vi "Test 2 Analog Sonar 3 MB7047 I2C Sensors.vi"() -> ()   [LabVIEW 2011]
uses:
  <vilib>/express/express arith-compare/Formula/XNode/ExpressFormulaBlockNode.xnode
  <vilib>/LabVIEW Interface for Arduino/LabVIEW Interface for Arduino.lvlib
panel:
  in  "Front Object\nDistance":i32=8
  out "Front Object":bool
  in  "Rear Object\nDistance":i32=3
  out "Rear Object":bool
  in  "Too Close\nto Manuver":i32=2
  out "Stop!":bool
  out "Turn Left":bool
  out "Right Front (ft)":dbl
  out "RF":dbl(slide) scale=0.0..10.0 scale format="%_4g"
  out "Left Front (ft)":dbl
  out "LF":dbl(slide) scale=0.0..10.0 scale format="%_4g"
  out "RB I2C Data":u8[](array[numeric]) format="%x"
  out "RB":u8(slide) scale=0.0..10.0
  out "Right Back (ft)":u32
  out "Center (ft)":u32
  out "C":u8(slide) scale=0.0..10.0
  out "C I2C Data":u8[](array[numeric]) format="%x"
  out "LB I2C Data":u8[](array[numeric]) format="%x"
  out "LB":u8(slide) scale=0.0..10.0
  out "Left Back (ft)":u32
  in  "stop":bool
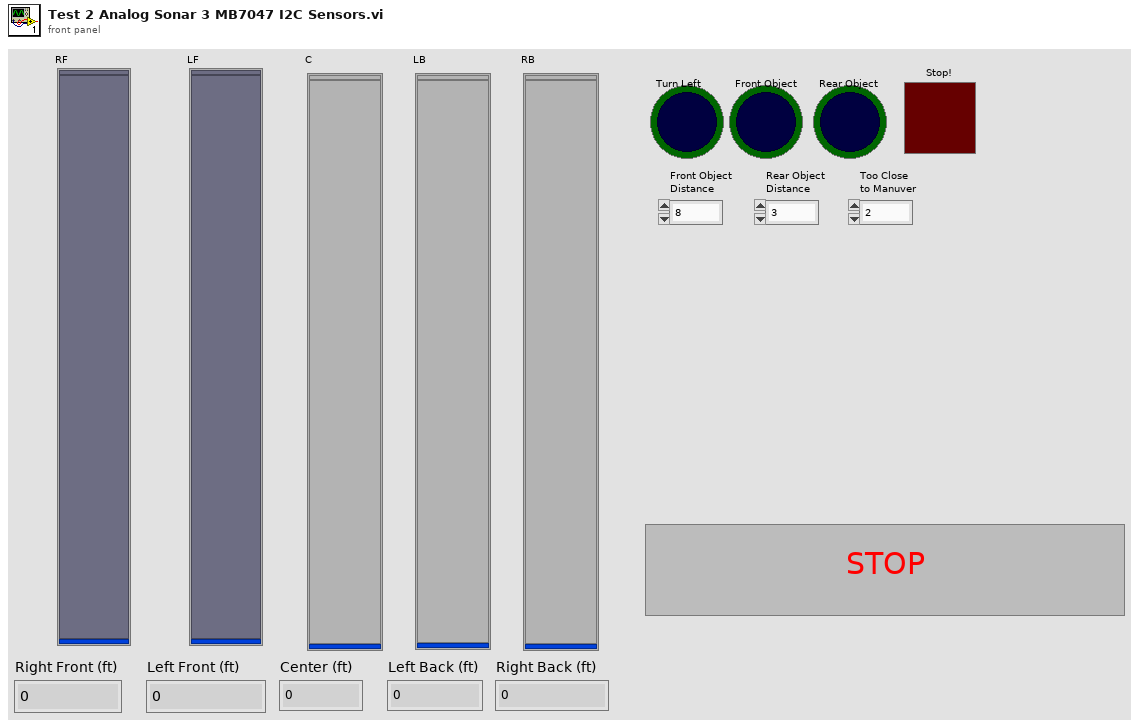
[diagram p1: front panel]
types:
  T1 = typedef "LabVIEW Interface for Arduino.lvlib/Arduino Resource.ctl" = cluster{"VISA resource":refnum<visa-resource-name>, "Board Type":T2, "Connection Type":enum8{"USB / Serial"}, "Bytes Per Packet (15)":u8}
  T2 = typedef "LabVIEW Interface for Arduino.lvlib/Board Type.ctl" = enum16{"Uno", "Dimuelanove w/Atmega 328", "Mega 2560"}
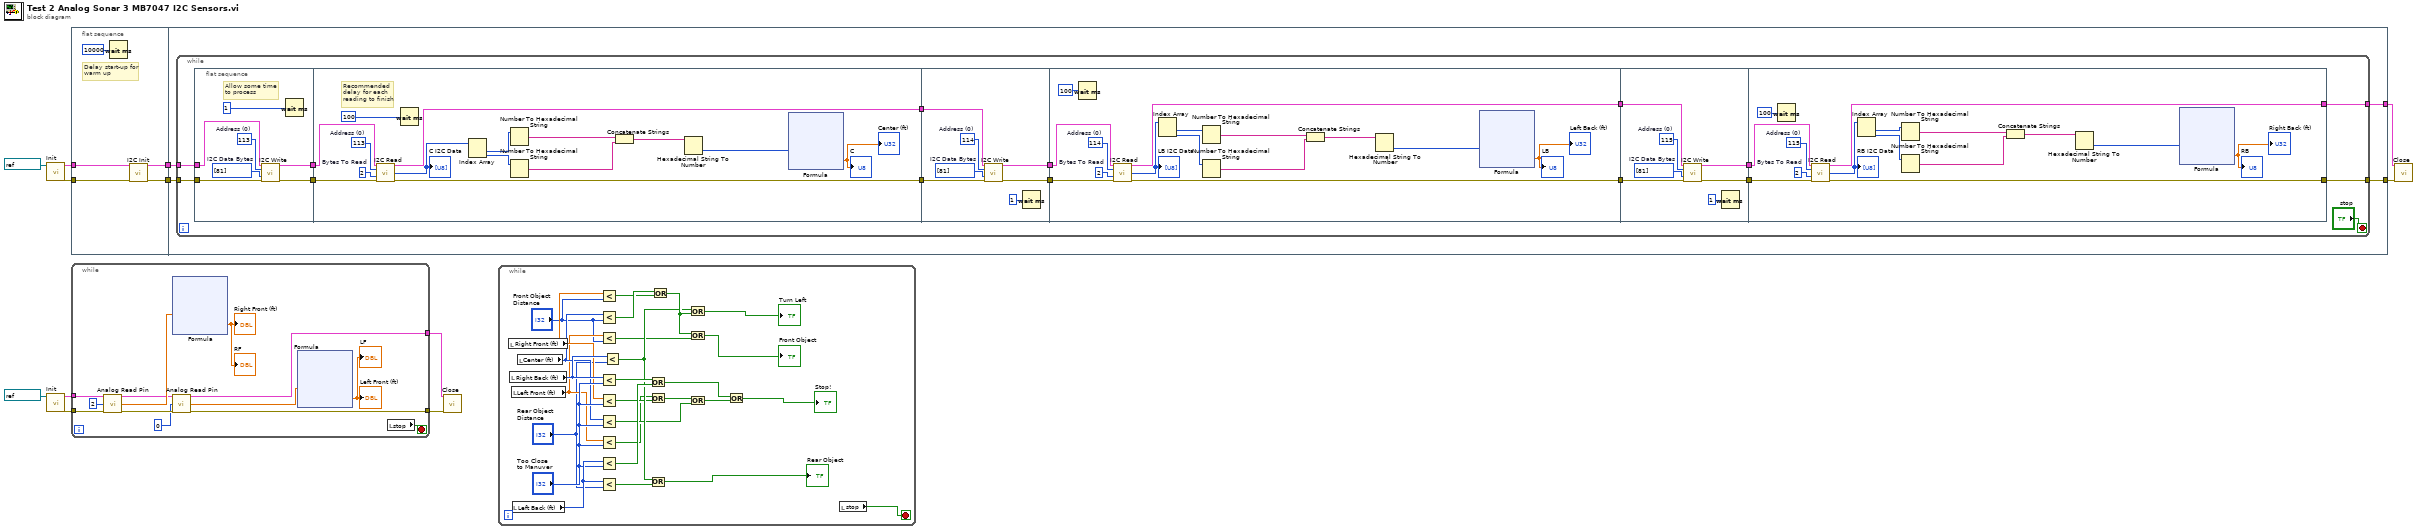
[diagram p0: block diagram]
diagram:
  n1 = call <vilib>:"Init.vi"("VISA resource"=refnum<visa-resource-name> "COM4") -> ("Arduino Resource"=w12:T1, "error out"=w11:errorcluster)  [unwired: 17 in]
  n2 = call <vilib>:"Init.vi"("VISA resource"=refnum<visa-resource-name> "COM6") -> ("Arduino Resource"=w9:T1, "error out"=w8:errorcluster)  [unwired: 17 in]
  n3 = flat-sequence {
    tunnel: w12 -> [w17]
    tunnel: w11 -> [w16]
    tunnel: [w15] -> w4
    tunnel: [w14] -> w3
    tunnel: w4 -> [w21]
    tunnel: w3 -> [w20]
    tunnel: [w19] -> w2
    tunnel: [w18] -> w1
    frame #0 {
      # "Delay start-up for\nwarm up"
      n4 = Wait (ms)(milliseconds to wait=u32 10000) -> ()  [unwired: 1 out]
      n5 = call <vilib>:"I2C Init.vi"("Arduino Resource"=w17, "error in"=w16) -> ("Arduino Resource"=w15:T1, "error out"=w14:errorcluster)  [unwired: 12 in]
    }
    frame #1 {
      n6 = while {
        tunnel: w21 -> [w36]
        tunnel: w20 -> [w35]
        tunnel: [w34] -> w18
        tunnel: [w33] -> w19
        stop <- "stop" stop-if-true
        n7 = flat-sequence {
          tunnel: [w43] -> w31
          tunnel: [w42] -> w30
          tunnel: w35 -> [w40]
          tunnel: w36 -> [w41]
          tunnel: [w58] -> w27
          tunnel: [w57] -> w26
          tunnel: w30 -> [w47]
          tunnel: w31 -> [w48]
          tunnel: [w73] -> w29
          tunnel: [w72] -> w28
          tunnel: w26 -> [w68]
          tunnel: w27 -> [w69]
          tunnel: [w88] -> w24
          tunnel: [w87] -> w23
          tunnel: w28 -> [w77]
          tunnel: w29 -> [w78]
          tunnel: [w103] -> w25
          tunnel: [w102] -> w22
          tunnel: w23 -> [w97]
          tunnel: w24 -> [w98]
          tunnel: w25 -> [w108]
          tunnel: w22 -> [w107]
          tunnel: [w109] -> w34
          tunnel: [w110] -> w33
          frame #0 {
            w39 = u8[] [81]  # I2C Data Bytes
            w38 = u8 113  # Address (0)
            # "Allow some time \nto process"
            n8 = call <vilib>:"I2C Write.vi"("Arduino Resource"=w41, "Address (0)"=w38, "I2C Data Bytes"=w39, "error in"=w40) -> ("Arduino Resource"=w43:T1, "error out"=w42:errorcluster)  [unwired: 10 in]
            n9 = Wait (ms)(milliseconds to wait=u32 1 ("Wait for Reading")) -> ()  [unwired: 1 out]
          }
          frame #1 {
            w49 = u8 113  # Address (0)
            w56 = u8 2  # Bytes To Read
            # "Recommended \ndelay for each \nreading to finish"
            n10 = call <vilib>:"I2C Read.vi"("Arduino Resource"=w48, "Address (0)"=w49, "Bytes To Read"=w56, "error in"=w47) -> ("Arduino Resource"=w58:T1, "I2C Data"=w50:u8[], "error out"=w57:errorcluster)  [unwired: 9 in]
            "C I2C Data" <- w50
            n11 = Wait (ms)(milliseconds to wait=u32 100 ("Delay (ms)")) -> ()  [unwired: 1 out]
            n12 = Index Array "Index Array"(array=w50) -> (element #1=w51:u8, element #2=w52:u8)  [unwired: 2 in]
            n13 = Number To Hexadecimal String(2:w51) -> (0:w54:string)  [unwired: 1 out]
            n14 = Number To Hexadecimal String(2:w52) -> (0:w53:string)  [unwired: 1 out]
            n15 = Concatenate Strings "Concatenate Strings"(w54, w53) -> (w55:string)
            n16 = Hexadecimal String To Number(string=w55) -> (number=w45:u32)  [unwired: 3 out]
            n17 = xnode "Formula"("cm"=w45) -> ("Result"=→"C" →"Center (ft)":dbl)  [unwired: 1 in, 1 out]
          }
          frame #2 {
            w70 = u8[] [81]  # I2C Data Bytes
            w71 = u8 114  # Address (0)
            n18 = call <vilib>:"I2C Write.vi"("Arduino Resource"=w69, "Address (0)"=w71, "I2C Data Bytes"=w70, "error in"=w68) -> ("Arduino Resource"=w73:T1, "error out"=w72:errorcluster)  [unwired: 10 in]
            n19 = Wait (ms)(milliseconds to wait=u32 1) -> ()  [unwired: 1 out]
          }
          frame #3 {
            w86 = u8 114  # Address (0)
            w79 = u8 2  # Bytes To Read
            n20 = Wait (ms)(milliseconds to wait=u32 100) -> ()  [unwired: 1 out]
            n21 = call <vilib>:"I2C Read.vi"("Arduino Resource"=w78, "Address (0)"=w86, "Bytes To Read"=w79, "error in"=w77) -> ("Arduino Resource"=w88:T1, "I2C Data"=w85:u8[], "error out"=w87:errorcluster)  [unwired: 9 in]
            "LB I2C Data" <- w85
            n22 = Index Array "Index Array"(array=w85) -> (element #1=w84:u8, element #2=w83:u8)  [unwired: 2 in]
            n23 = Number To Hexadecimal String(2:w84) -> (0:w81:string)  [unwired: 1 out]
            n24 = Number To Hexadecimal String(2:w83) -> (0:w82:string)  [unwired: 1 out]
            n25 = Concatenate Strings "Concatenate Strings"(w81, w82) -> (w80:string)
            n26 = Hexadecimal String To Number(string=w80) -> (number=w75:u32)  [unwired: 3 out]
            n27 = xnode "Formula"("cm"=w75) -> ("Result"=→"LB" →"Left Back (ft)":dbl)  [unwired: 1 in, 1 out]
          }
          frame #4 {
            w99 = u8[] [81]  # I2C Data Bytes
            w100 = u8 115  # Address (0)
            n28 = call <vilib>:"I2C Write.vi"("Arduino Resource"=w98, "Address (0)"=w100, "I2C Data Bytes"=w99, "error in"=w97) -> ("Arduino Resource"=w102:T1, "error out"=w103:errorcluster)  [unwired: 10 in]
            n29 = Wait (ms)(milliseconds to wait=u32 1) -> ()  [unwired: 1 out]
          }
          frame #5 {
            w111 = u8 115  # Address (0)
            w118 = u8 2  # Bytes To Read
            n30 = Wait (ms)(milliseconds to wait=u32 100) -> ()  [unwired: 1 out]
            n31 = call <vilib>:"I2C Read.vi"("Arduino Resource"=w107, "Address (0)"=w111, "Bytes To Read"=w118, "error in"=w108) -> ("Arduino Resource"=w109:T1, "I2C Data"=w112:u8[], "error out"=w110:errorcluster)  [unwired: 9 in]
            "RB I2C Data" <- w112
            n32 = Index Array "Index Array"(array=w112) -> (element #1=w113:u8, element #2=w114:u8)  [unwired: 2 in]
            n33 = Number To Hexadecimal String(2:w113) -> (0:w116:string)  [unwired: 1 out]
            n34 = Number To Hexadecimal String(2:w114) -> (0:w115:string)  [unwired: 1 out]
            n35 = Concatenate Strings "Concatenate Strings"(w116, w115) -> (w117:string)
            n36 = Hexadecimal String To Number(string=w117) -> (number=w105:u32)  [unwired: 3 out]
            n37 = xnode "Formula"("cm"=w105) -> ("Result"=→"RB" →"Right Back (ft)":dbl)  [unwired: 1 in, 1 out]
          }
        }
      }
    }
  }
  n38 = while {
    tunnel: w9 -> [w139]
    tunnel: w8 -> [w138]
    tunnel: [w131] -> w6
    tunnel: [w130] -> w5
    stop <- w127 stop-if-true
    n39 = call <vilib>:"Analog Read Pin.vi"("Arduino Resource"=w139, "Analog Input Pin (0)"=u8 2, "error in"=w138) -> ("Arduino Resource"=w135:T1, "Voltage"=w136:dbl, "error out"=w134:errorcluster)  [unwired: 10 in]
    n40 = xnode "Formula"("Vin"=w136) -> ("Result"=→"Right Front (ft)" →"RF":dbl)  [unwired: 1 in, 1 out]
    n41 = call <vilib>:"Analog Read Pin.vi"("Arduino Resource"=w135, "Analog Input Pin (0)"=u8 0, "error in"=w134) -> ("Arduino Resource"=w130:T1, "Voltage"=w132:dbl, "error out"=w131:errorcluster)  [unwired: 10 in]
    n42 = xnode "Formula"("Vin"=w132) -> ("Result"=→"Left Front (ft)" →"LF":dbl)  [unwired: 1 in, 1 out]
    n43 = local read "stop"() -> (w127:bool)
  }
  n44 = call <vilib>:"Close.vi"("Arduino Resource"=w5, "error in"=w6) -> ()  [unwired: 13 in, 1 out]
  n45 = while {
    stop <- w156 stop-if-true
    n46 = local read "Right Front (ft)"() -> (w163:dbl)
    n47 = local read "Right Back (ft)"() -> (w177:u32)
    n48 = local read "Left Front (ft)"() -> (w162:dbl)
    n49 = local read "Left Back (ft)"() -> (w176:u32)
    n50 = local read "Center (ft)"() -> (w164:u32)
    n51 = Less?(x=w163, y="Front Object\nDistance") -> (x < y?=w158:bool)
    n52 = Less?(x=w164, y="Front Object\nDistance") -> (x < y?=w171:bool)
    n53 = Less?(x=w162, y="Front Object\nDistance") -> (x < y?=w170:bool)
    n54 = Less?(x=w177, y="Too Close\nto Manuver") -> (x < y?=w178:bool)
    n55 = Less?(x=w163, y="Too Close\nto Manuver") -> (x < y?=w166:bool)
    n56 = Less?(x=w164, y="Too Close\nto Manuver") -> (x < y?=w167:bool)
    n57 = Less?(x=w162, y="Too Close\nto Manuver") -> (x < y?=w165:bool)
    n58 = Less?(x=w176, y="Too Close\nto Manuver") -> (x < y?=w179:bool)
    n59 = Less?(x=w176, y="Rear Object\nDistance") -> (x < y?=w169:bool)
    n60 = Less?(x=w177, y="Rear Object\nDistance") -> (x < y?=w172:bool)
    n61 = Or(x=w178, y=w179) -> (x .or. y?=w180:bool)
    n62 = Or(x=w165, y=w166) -> (x .or. y?=w168:bool)
    n63 = Or(x=w172, y=w169) -> (x .or. y?=→"Rear Object":bool)
    n64 = Or(x=w171, y=w158) -> (x .or. y?=w173:bool)
    n65 = Or(x=w172, y=w173) -> (x .or. y?=→"Turn Left":bool)
    n66 = Or(x=w173, y=w170) -> (x .or. y?=→"Front Object":bool)
    n67 = Or(x=w168, y=w167) -> (x .or. y?=w181:bool)
    n68 = Or(x=w180, y=w181) -> (x .or. y?=→"Stop!":bool)
    n69 = local read "stop"() -> (w156:bool)
  }
  n70 = call <vilib>:"Close.vi"("Arduino Resource"=w1, "error in"=w2) -> ()  [unwired: 13 in, 1 out]
